vi "SM_S700_Serial_Parser.vi"(0 "co2 in":dbl, 1 "ch4 in":dbl, 2 "read buffer":string, 5 "h2 in":dbl, 7 "pump in":bool, 11 "error in (no error)":errorcluster, 12 "timestamp in":timestamp) -> (3 "timestamp out":timestamp, 4 "ch4 out":dbl, 6 "co2 out":dbl, 8 "h2 out":dbl, 10 "pump out":bool, 15 "error out":errorcluster)   [LabVIEW 2011]
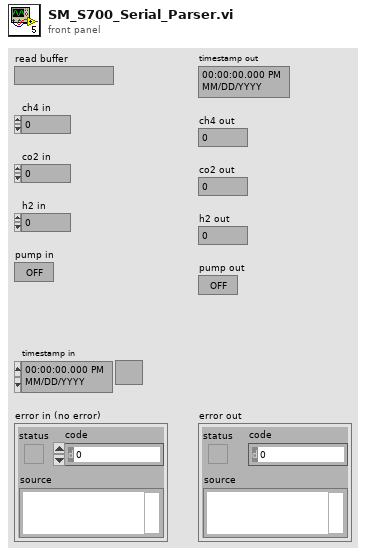
[diagram p1: front panel]
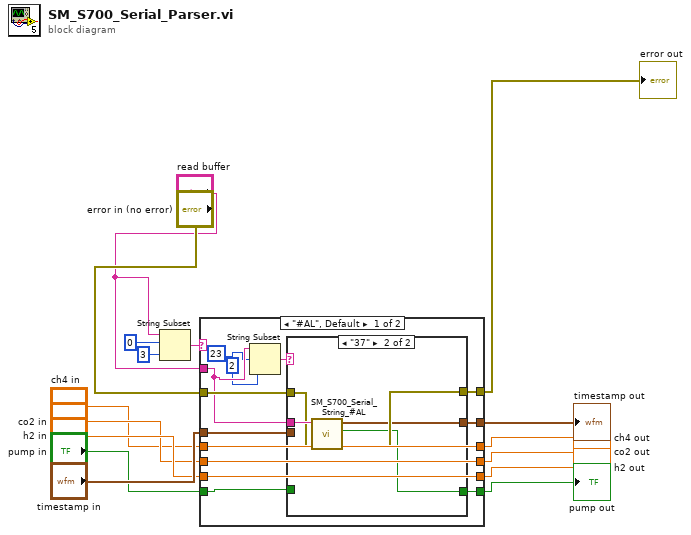
[diagram p0: block diagram]
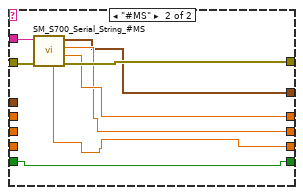
[diagram p3: hidden frame]
diagram:
  n1 = String Subset(string="read buffer", offset (0)=0, length (rest)=3 ("length (rest)")) -> (substring=w2:string)
  n2 = case shown="\"#AL\", Default" w2 {
    tunnel: "error in (no error)" -> [w29 w45]
    tunnel: [w28 w44] -> w10
    tunnel: "read buffer" -> [w27 w43]
    tunnel: "ch4 in" -> [w25 _]
    tunnel: "co2 in" -> [w24 _]
    tunnel: "h2 in" -> [w23 _]
    tunnel: "pump in" -> [w22 w39]
    tunnel: [w25 w42] -> w11
    tunnel: [w24 w41] -> w12
    tunnel: [w23 w40] -> w13
    tunnel: [w21 w39] -> w14
    tunnel: [w18 w38] -> w15
    tunnel: "timestamp in" -> [w17 _]
    frame "#AL", Default {
      n3 = String Subset(string=w27, offset (0)=23, length (rest)=2 ("length (rest)")) -> (substring=w20:string)
      n4 = case shown="\"37\"" w20 {
        tunnel: w27 -> [_ w37]
        tunnel: w29 -> [w32 w36]
        tunnel: [w32 w35] -> w28
        tunnel: w22 -> [w31 _]
        tunnel: [w31 w34] -> w21
        tunnel: [w30 w33] -> w18
        tunnel: w17 -> [w30 _]
        frame Default {
        }
        frame "37" {
          n5 = call "SM_S700_Serial_String_#AL.vi"("error in (no error)"=w36, "read buffer"=w37) -> ("error out"=w35:errorcluster, "pump"=w34:bool, "timestamp"=w33:timestamp)  [unwired: 7 in]
        }
      }
    }
    frame "#MS" {
      n6 = call "SM_S700_Serial_String_#MS.vi"("error in (no error)"=w45, "read buffer"=w43) -> ("error out"=w44:errorcluster, "ch4"=w42:dbl, "co2"=w41:dbl, "timestamp"=w38:timestamp, "h2"=w40:dbl)  [unwired: 5 in]
    }
  }
  "timestamp out" <- w15
  "pump out" <- w14
  "h2 out" <- w13
  "co2 out" <- w12
  "ch4 out" <- w11
  "error out" <- w10
